vi "svfa_Average Array with Avg Checks (complex) No State.vi"(0 "spectrum":cdb[](array[numeric]) format="%.2p", 1 "processing control":T1(ring), 11 "error in (no error)":errorcluster, 12 "averaging state info in":T2={"complex FFT"=[], "real FFT"=[], "f0"=0.0, "df"=0.0, "averages completed"=0.0, "averaging parameters"={"averaging mode"=enum."No averaging", "weighting mode"=enum."Linear", "number of averages"=10, "linear mode"=enum."Auto restart"}} {"averages completed" format="%.2f"; "df" format="%.2f"; "f0" format="%.2f"; "real FFT" format="%.2f"; "complex FFT" format="%.2f"}) -> (4 "average spectrum":cdb[](array[numeric]) format="%.2p", 6 "new spectrum ready":bool, 8 "averaging done":bool, 10 "averages completed":dbl, 14 "averaging state info out":T2={"complex FFT"=[], "real FFT"=[], "f0"=0.0, "df"=0.0, "averages completed"=0.0, "averaging parameters"={"averaging mode"=enum."No averaging", "weighting mode"=enum."Linear", "number of averages"=10, "linear mode"=enum."Auto restart"}} {"averages completed" format="%.2f"; "df" format="%.2f"; "f0" format="%.2f"; "real FFT" format="%.2f"; "complex FFT" format="%.2f"}, 15 "error out":errorcluster)   [LabVIEW 2017]
uses:
  <vilib>/addons/_NISVFA/_Shared subVIs/Spectrum Averaging/svfa_No Average Array (complex).vi
  <vilib>/addons/_NISVFA/_Shared subVIs/Spectrum Averaging/svfa_Average Array (complex).vi
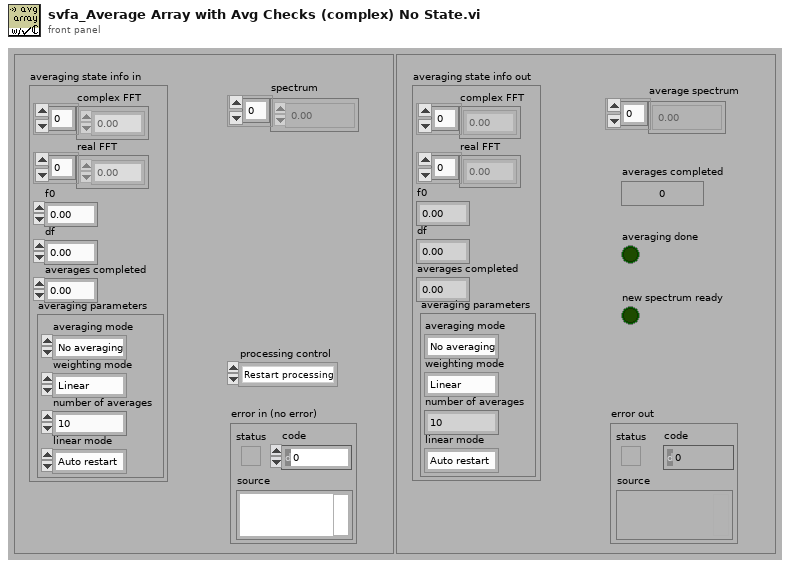
[diagram p1: front panel]
types:
  T1 = enum16{"Restart processing", "Continue processing", "Skip processing"}
  T2 = cluster{"complex FFT":cdb[], "real FFT":dbl[], "f0":dbl, "df":dbl, "averages completed":dbl, "averaging parameters":cluster{"averaging mode":enum16{"No averaging", "Vector averaging", "RMS averaging", "Peak hold"}, "weighting mode":enum16{"Linear", "Exponential"}, "number of averages":u32, "linear mode":enum16{"One shot", "Auto restart"}}}
  T3 = cluster{"complex FFT":cdb[], "Mag/Real FFT":dbl[], "f0":dbl, "df":dbl, "averages completed":dbl, "averaging parameters":cluster{"averaging mode":enum16{"No averaging", "Vector averaging", "RMS averaging", "Peak hold"}, "weighting mode":enum16{"Linear", "Exponential"}, "number of averages":u32, "linear mode":enum16{"One shot", "Auto restart"}}}
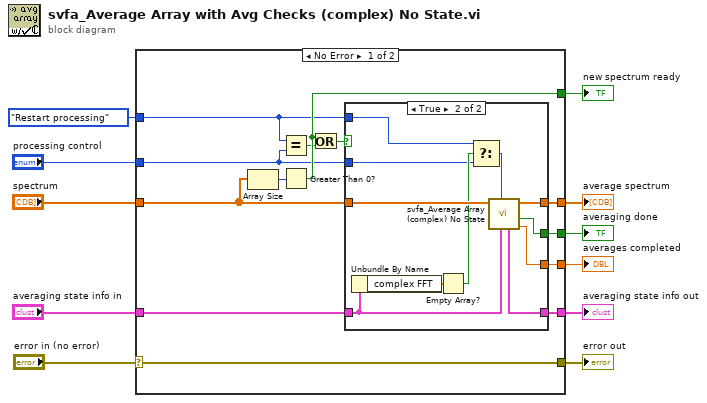
[diagram p0: block diagram]
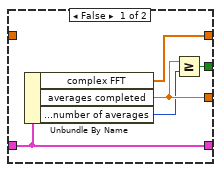
[diagram p2: hidden frame]
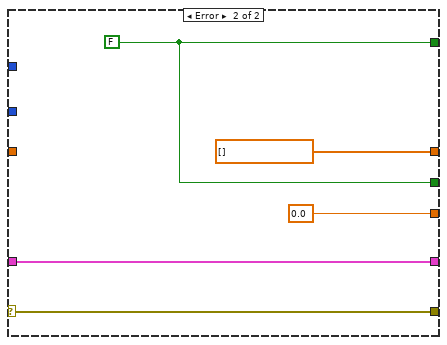
[diagram p3: hidden frame]
diagram:
  n1 = case shown="No Error" "error in (no error)" {
    selector: "error in (no error)" -> [w14 w41]
    tunnel: "spectrum" -> [w15 _]
    tunnel: [w23 cdb[] []] -> w10
    tunnel: [w22 w42] -> w9
    tunnel: [w20 w45] -> w8
    tunnel: "averaging state info in" -> [w19 w42]
    tunnel: "processing control" -> [w13 _]
    tunnel: [w17 0.0 ("averages completed")] -> w6
    tunnel: [w16 w45] -> w5
    tunnel: [w14 w41] -> w3
    tunnel: T1."Restart processing" ("processing control") -> [w12 _]
    frame No Error {
      n2 = Array Size(array=w15) -> (size(s)=w24:i32)
      n3 = Equal?(x=w12, y=w13) -> (x = y?=w18:bool)
      n4 = Greater Than 0?(x=w24) -> (x > 0?=w20:bool)
      n5 = Or(x=w20, y=w18) -> (x .or. y?=w21:bool)
      n6 = case shown="True" w21 {
        tunnel: [w26 w38] -> w23
        tunnel: [w27 w40] -> w17
        tunnel: w19 -> [w28 w35]
        tunnel: [w28 w39] -> w22
        tunnel: w13 -> [_ w31]
        tunnel: [w29 w37] -> w16
        tunnel: w15 -> [_ w36]
        tunnel: w12 -> [_ w33]
        frame False {
          n7 = Unbundle By Name(w28) -> ("complex FFT"=w26:cdb[], "averages completed"=w27:dbl, "averaging parameters.number of averages"=w25:u32)
          n8 = Greater Or Equal?(x=w27, y=w25) -> (x >= y?=w29:bool)
        }
        frame True {
          n9 = Unbundle By Name(w35) -> ("complex FFT"=w34:cdb[])
          n10 = Empty Array?(array=w34) -> (empty?=w32:bool)
          n11 = Select(t=w33, s=w32, f=w31) -> (s? t:f=w30:T1)
          n12 = call <vilib>:"svfa_Average Array (complex) No State.vi"("averaging state info in"=w35, "processing control"=w30, "array"=w36) -> ("averages completed"=w40:dbl, "averaging done"=w37:bool, "average array"=w38:cdb[], "averaging state info out"=w39:T3)  [unwired: 5 in]
        }
      }
    }
    frame Error {
      w45 = FALSE
    }
  }
  "average spectrum" <- w10
  "averaging state info out" <- w9
  "averages completed" <- w6
  "new spectrum ready" <- w8
  "averaging done" <- w5
  "error out" <- w3
